vi "S2C_ExeBreakOnFailOps.vi"(8 "Error In":errorcluster, 10 "LastStep?":bool, 11 "Q_Ref":refnum<queue>) -> (0 "Error Out":errorcluster, 3 "IncRow?":bool)   [LabVIEW 2015]
doc: "Update the results cell in the execution table for the currently executing line item, and determines the next step to take in the execution."
uses:
  Globals/S2C_Globals.vi
panel:
  in  "Text":string="A test failure has occurred while \"Break on Failure\" was active.\n\nWhat would you like to do?"
  in  "Abort":bool
  in  "Continue":bool
  in  "Retest":bool
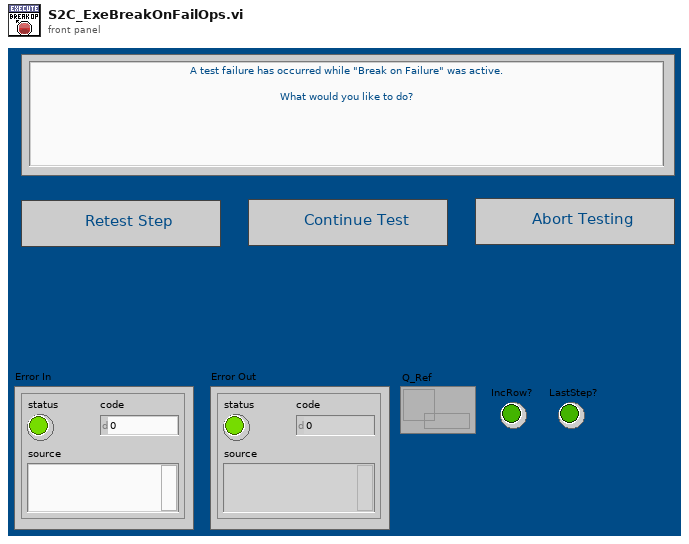
[diagram p1: front panel]
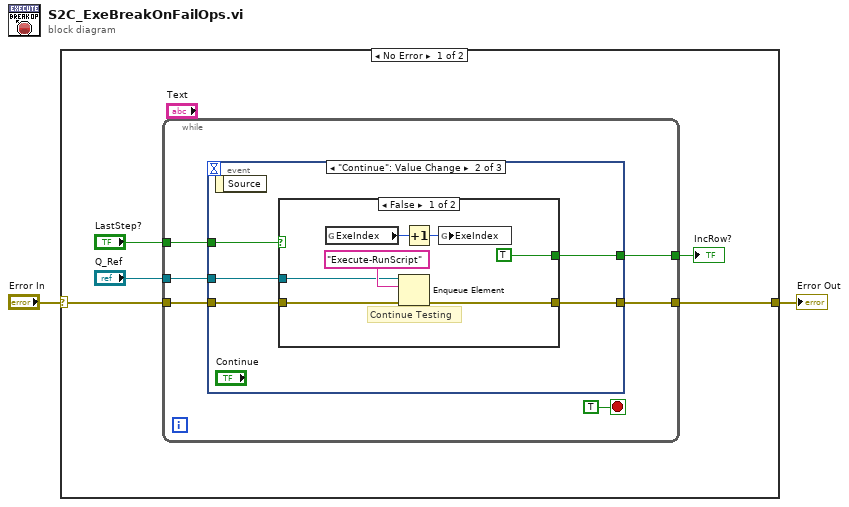
[diagram p0: block diagram]
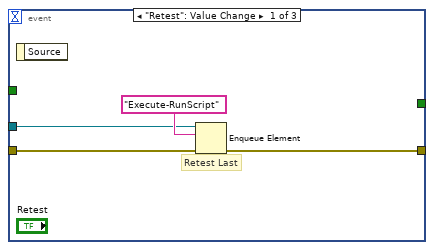
[diagram p2: hidden frame]
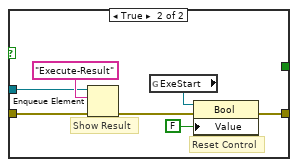
[diagram p3: hidden frame]
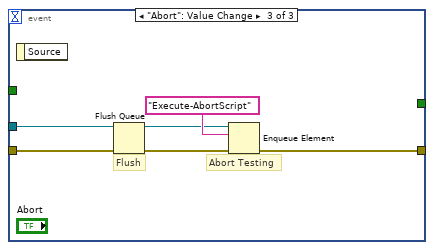
[diagram p4: hidden frame]
diagram:
  n1 = case shown="No Error" "Error In" {
    selector: "Error In" -> [w7 w43]
    tunnel: [w6 w43] -> w1
    frame No Error {
      n2 = while {
        tunnel: w7 -> [w13]
        tunnel: [w12] -> w6
        tunnel: "Q_Ref" -> [w11]
        tunnel: [w9] -> w4
        tunnel: "LastStep?" -> [w8]
        stop <- TRUE stop-if-true
        n3 = event shown="[1] \"Continue\": Value Change" {
          selector: _ -> [_ _ _]
          dyn-events: _ -> [_ _ _]
          timeout: _ -> [_ _ _]
          tunnel: w13 -> [w15 w22 w39]
          tunnel: [w14 w21 w38] -> w12
          tunnel: w11 -> [w16 w20 w37]
          tunnel: [_ w19 _] -> w9
          tunnel: w8 -> [_ w18 _]
          event "Retest": Value Change {
            # "Retest Last"
            n4 = event-data() -> ()  [unwired: 1 in, 1 out]
            n5 = Enqueue Element(queue=w16, element="Execute-RunScript", error in (no error)=w15) -> (error out=w14:errorcluster)  [unwired: 1 in, 2 out]
          }
          event "Continue": Value Change {
            n6 = event-data() -> ()  [unwired: 1 in, 1 out]
            n7 = case shown="False" w18 {
              tunnel: w22 -> [w27 w32]
              tunnel: [w26 w30] -> w21
              tunnel: w20 -> [w25 w31]
              tunnel: [TRUE _] -> w19
              frame False {
                # "Continue Testing"
                n8 = global read "S2C_Globals.vi" "ExeIndex"() -> (w24:i32)
                n9 = Enqueue Element(queue=w25, element="Execute-RunScript", error in (no error)=w27) -> (error out=w26:errorcluster)  [unwired: 1 in, 2 out]
                n10 = Increment(x=w24) -> (x+1=w28:i32)
                n11 = global write "S2C_Globals.vi" "ExeIndex"(w28) -> ()
              }
              frame True {
                # "Show Result"
                # "Reset Control"
                n12 = Enqueue Element(queue=w31, element="Execute-Result", error in (no error)=w32) -> (error out=w35:errorcluster)  [unwired: 1 in, 2 out]
                n13 = global read "S2C_Globals.vi" "ExeStart"() -> (w33:refnum<vi>)
                n14 = property class="Bool"(reference=w33, error in=w35, "Value"=FALSE) -> (error out=w30:errorcluster)  [unwired: 1 out]
              }
            }
          }
          event "Abort": Value Change {
            # "Flush"
            # "Abort Testing"
            n15 = event-data() -> ()  [unwired: 1 in, 1 out]
            n16 = Flush Queue(queue=w37, error in (no error)=w39) -> (queue out=w40:refnum<queue>, error out=w41:errorcluster)  [unwired: 1 out]
            n17 = Enqueue Element(queue=w40, element="Execute-AbortScript", error in (no error)=w41) -> (error out=w38:errorcluster)  [unwired: 1 in, 2 out]
          }
        }
      }
      "IncRow?" <- w4
    }
    frame Error {
    }
  }
  "Error Out" <- w1
